vi "shift_data(waveform).vi"(9 "value":sgl, 10 "篇移位數":i32=-1, 11 "Array":sgl[](array[numeric])) -> (3 "Waveform":sgl[](graph))   [LabVIEW 2019]
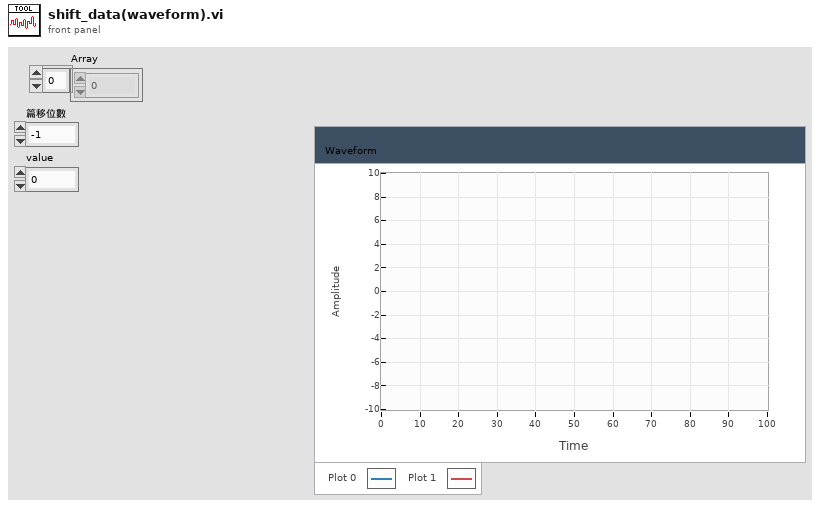
[diagram p1: front panel]
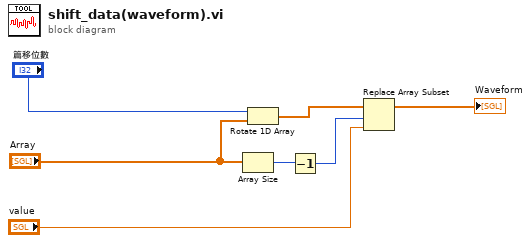
[diagram p0: block diagram]
diagram:
  n1 = Array Size(array="Array") -> (size(s)=w3:i32)
  n2 = Rotate 1D Array(1:"Array", 2:"篇移位數") -> (0:w6:sgl[])
  n3 = Decrement(x=w3) -> (x-1=w2:i32)
  n4 = Replace Array Subset(array=w6, new element="value", index=w2) -> (→"Waveform":sgl[])
